vi "FlatSequenceExample.vi"() -> ()   [LabVIEW 2018]
panel:
  in  "Y":dbl
  in  "X":dbl
  out "X + Y =":dbl
  in  "Compute X + Y":bool
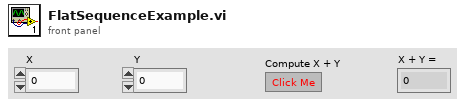
[diagram p1: front panel]
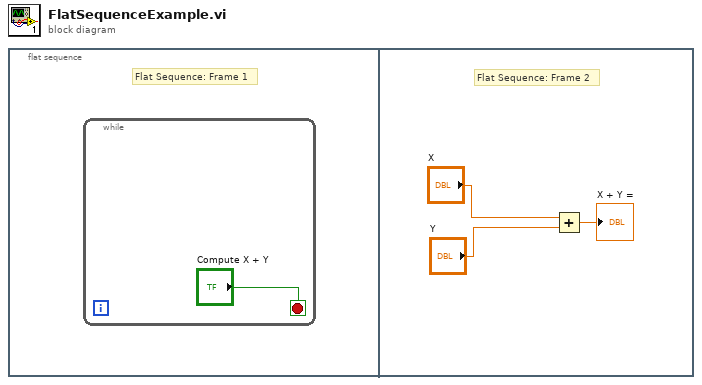
[diagram p0: block diagram]
diagram:
  n1 = flat-sequence {
    frame #0 {
      # "Flat Sequence: Frame 1"
      n2 = while {
        stop <- "Compute X + Y" stop-if-true
      }
    }
    frame #1 {
      # "Flat Sequence: Frame 2"
      n3 = Add(x="X", y="Y") -> (x+y=→"X + Y =":dbl)
    }
  }
